vi "SensorRefNums.vi"() -> (0 "Sensors":T1)   [LabVIEW 2018]
uses:
  TypeDefs/RobotComponents/RobotSensors.ctl
  ArgosLib/Config/ConfigComponents/TypeDefs/Config_DigitalIO.ctl
  <vilib>/Rock Robotics/SystemInterfaces/DIO/FPGA_DIOChannel.ctl
  ArgosLib/ArgosLib.lvlib
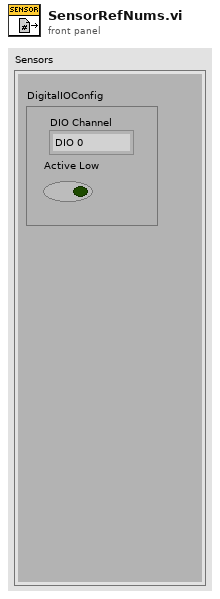
[diagram p1: front panel]
types:
  T1 = typedef "RobotSensors.ctl" = cluster{"DigitalIOConfig":T2}
  T2 = typedef "ArgosLib.lvlib/Config_DigitalIO.ctl" = cluster{"DIOChannel":T3, "Active Low":bool}
  T3 = typedef "FPGA_DIOChannel.ctl" = enum8{"DIO 0", "DIO 1", "DIO 2", "DIO 3", "DIO 4", "DIO 5", "DIO 6", "DIO 7", "DIO 8", "DIO 9", "DIO MXP 0", "DIO MXP 1", "DIO MXP 2", "DIO MXP 3", "DIO MXP 4", "DIO MXP 5", "DIO MXP 6", "DIO MXP 7", "DIO MXP 8", "DIO MXP 9", "DIO MXP 10", "DIO MXP 11", "DIO MXP 12", "DIO MXP 13", "DIO MXP 14", "DIO MXP 15", "SPI Port CS1", "SPI Port CS2", "SPI Port CS3", "SPI Port MISO", "SPI Port MOSI", "Invalid"}
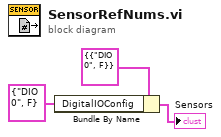
[diagram p0: block diagram]
diagram:
  n1 = Bundle By Name(cluster=T1 {"DigitalIOConfig"={"DIOChannel"=enum."DIO 0", "Active Low"=FALSE}} ("Sensors"), "DigitalIOConfig"=T2 {"DIOChannel"=enum."DIO 0", "Active Low"=FALSE}) -> (→"Sensors":T1)
